vi "Flatten to CSV Record.vi"(0 "row of strings":string[](array[string]), 1 "protected symbol (,)":string=",", 2 "item separator (empty - use protected symbol)":string, 5 "error in (no error)":errorcluster) -> (3 "can be indented?":bool, 4 "CSV record":string, 6 "error out":errorcluster)   [LabVIEW 2013, in "infolib.lvlib"]
doc: "Convert 1D array of ANSI strings into a single CSV record (row or column).\n\nThe output CSV record string is formatted in accordance with RFC-4180 (see <b>http://tools.ietf.org/html/rfc4180<\\b>). \n\nAll cells containing double quotes (0x22), CR (0x0D) , LF (0x0A) or the delimiter character will be enclosed in double quotes. All double quote characters within a cell will be escaped using a second double quote character.\n\nRev. 0.0 2014-02-20 Ryan Porter\n- First Draft\n\nRev 0.1 2014-10-30 Ryan Porter\n- Convert all CRLF and CR within a cell to LF\n- Changed end of record to CRLF for compatibility with Excel CSV import/export\n\nRev 0.2 2017-01-03 modified for infolib\n\nRev 0.3 2017-01-20 can generate also column vector"
uses:
  infolib.lvlib
panel:
  # "Flatten to CSV Record.vi\n\nConvert 1D array of ANSI strings into a single CSV record (row). The output CSV record string is formatted in accordance with RFC-4180 (see http://tools.ietf.org/html/rfc4180). \n\nAll cells containing double quotes (0x22), CR (0x0D) , LF (0x0A) or the delimiter character will be enclosed in double quotes. All double quote characters within a cell will be escaped using a second double quote character. A CRLF is appended to the end of the record."
  # "License: BSD (2-Clause) - http://opensource.org/licenses/BSD-2-Clause \n\nCopyright (c) 2014, Ryan Porter\nAll rights reserved."
  # "Robust CSV v1.1.0\n\nCopyright © 2014, Ryan Porter\nAll rights reserved.\n\nAuthor:\t Ryan Porter\nLAVA Name: Porter\nContact Info:\tContact via PM on lavag.org\n\nLabVIEW Versions:\nLV 2013 (Windows)\nLV 2012 (Windows)\nLV 8.6 (Windows)\n\nDependencies:\nLAVA Palette\n\nDescription:\nThis package contains VIs for reading and writing to CSV files that follow the CSV format outlined in RFC-4180 (see http://tools.ietf.org/html/rfc4180). Using this package, you can properly import CSV files that were exported from spreadsheet programs such as Microsoft Excel, Open Office or LibreOffice Calc as well as export CSV files that will be compatible with any program capable of interpreting CSV files.\n \nThis implementation of the CSV format is capable of handling escaped fields such as those containing commas (or other field delimiters), multiple lines, and double quotes.\n\nInstallation and instructions:\nInstall VIP package using JKI VI Package Manager.\n\nExamples:\n\"<LabVIEW>\\examples\\LAVA\\Robust CSV\\Robust CSV Example Usage.vi\"\tDemonstrates usage of the Read CSV and Write CSV file.\n\nKnown Issues:\nnone\n\nAcknowledgements:\nPhillip Brooks: \"Parse CSV String.vi\" is a modified version of his \"CSV Data File Parser.vi\". His method of parsing the CSV string was much more efficient than my original implementation.\n\nVersion History:\nv1.0.0: Initial release of the code.\nv1.0.1: Modified \"Flatten to CSV Record.vi\" to play nice with Excel CSV import when multi-line cells are present.\nv1.1.0: Moved to LAVA palette & built to VI package file.\n\nLicense:\nDistributed under the BSD 2-Clause (http://opensource.org/licenses/BSD-2-Clause)\nSee link for a full description of the license.\n\nSupport:\nIf you have any problems with this code or want to suggest features go to lavag.org and Navigate to LAVA > Resources > Code Repository (Certified) and\nsearch for the \"Robust CSV\" support page. Or try this link: http://lavag.org/files/file/239-robust-csv/\n\nDistribution:\nThis code was downloaded from the LAVA Code Repository found at lavag.org"
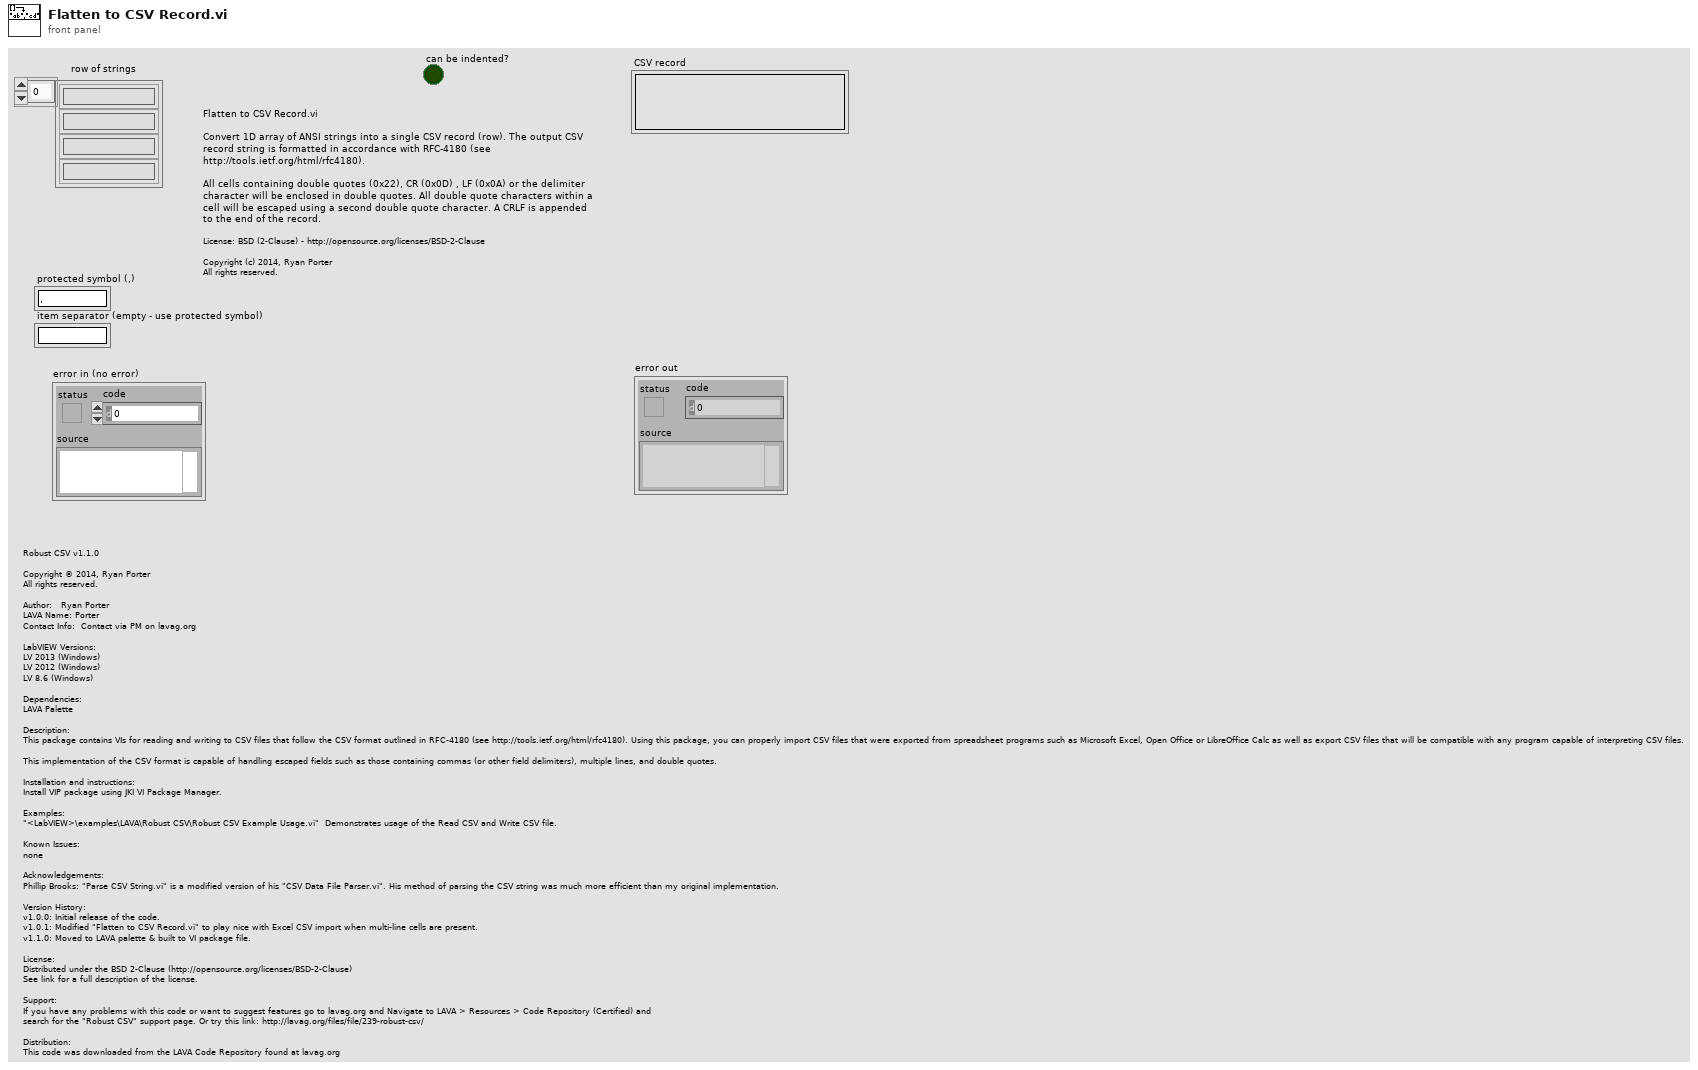
[diagram p1: front panel]
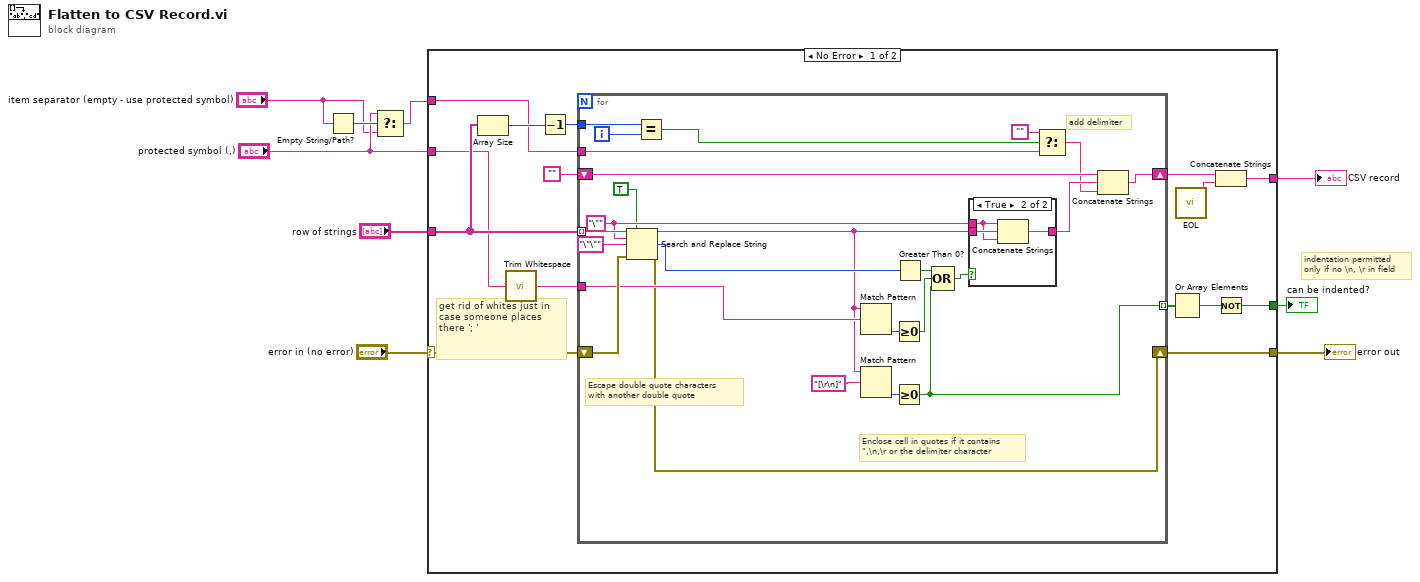
[diagram p0: block diagram]
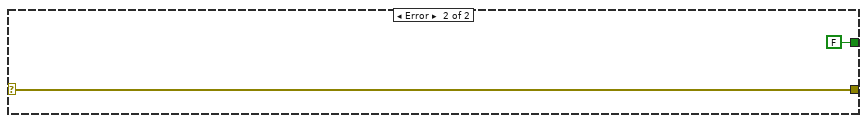
[diagram p3: hidden frame]
diagram:
  # "indentation permitted\nonly if no \\n, \\r in field"
  n1 = Empty String/Path?(string/path="item separator (empty - use protected symbol)") -> (empty?=w4:bool)
  n2 = Select(t="protected symbol (,)", s=w4, f="item separator (empty - use protected symbol)") -> (s? t:f=w1:string)
  n3 = case shown="No Error" "error in (no error)" {
    selector: "error in (no error)" -> [w18 w55]
    tunnel: "row of strings" -> [w22 _]
    tunnel: "protected symbol (,)" -> [w15 _]
    tunnel: [w19 _] -> w8
    tunnel: [w17 w55] -> w6
    tunnel: [w12 FALSE] -> w5
    tunnel: w1 -> [w10 _]
    frame No Error {
      # "get rid of whites just in case someone places there '; '"
      n4 = Array Size(array=w22) -> (size(s)=w21:i32)
      n5 = call <vilib>:"Trim Whitespace.vi"("string"=w15) -> ("trimmed string"=w11:string)  [unwired: 1 in]
      n6 = Decrement(x=w21) -> (x-1=w23:i32)
      n7 = for {
        tunnel: w22 -> [w49] mode=indexing
        shift-right: [w46] -> w20
        shift-left: "" -> [w45]
        tunnel: w10 -> [w40]
        tunnel: w23 -> [w37]
        shift-right: [w28] -> w17
        shift-left: w18 -> [w34]
        tunnel: [w25] -> w16 mode=indexing
        tunnel: w11 -> [w29]
        i -> [w42]
        w47 = "\"" ("search string")
        # "Escape double quote characters\nwith another double quote"
        # "Enclose cell in quotes if it contains\n\",\\n,\\r or the delimiter character"
        # "add delimiter"
        n8 = Search and Replace String(replace all?=TRUE ("replace all? (F)"), input string=w49, search string=w47, replace string="\"\"" ("replace string (\"\")"), error in=w34) -> (result string=w27:string, number of replacements=w36:i32, error out=w28:errorcluster)  [unwired: 4 out]
        n9 = Equal?(x=w37, y=w42) -> (x = y?=w41:bool)
        n10 = Match Pattern(string=w27, regular expression=w29) -> (offset past match=w43:i32)  [unwired: 4 out]
        n11 = Match Pattern(string=w27, regular expression="[\r\n]") -> (offset past match=w31:i32)  [unwired: 4 out]
        n12 = Greater Or Equal To 0?(x=w43) -> (x >= 0?=w26:bool)
        n13 = Greater Or Equal To 0?(x=w31) -> (x >= 0?=w25:bool)
        n14 = Greater Than 0?(x=w36) -> (x > 0?=w32:bool)
        n15 = Compound Arithmetic op=OR(w32, w26, w25) -> (w35:bool)
        n16 = case shown="True" w35 {
          tunnel: w27 -> [w50 w53]
          tunnel: w47 -> [_ w52]
          tunnel: [w50 w51] -> w44
          frame False {
          }
          frame True {
            n17 = Concatenate Strings(w52, w53, w52) -> (w51:string)
          }
        }
        n18 = Select(t="", s=w41, f=w40) -> (s? t:f=w38:string)
        n19 = Concatenate Strings(w45, w44, w38) -> (w46:string)
      }
      n20 = Or Array Elements(Boolean array=w16) -> (logical OR=w13:bool)
      n21 = call "EOL.vi"() -> ("eol"=w14:string)  [unwired: 11 in]
      n22 = Concatenate Strings(w20, w14) -> (w19:string)
      n23 = Not(x=w13) -> (.not. x?=w12:bool)
    }
    frame Error {
    }
  }
  "CSV record" <- w8
  "error out" <- w6
  "can be indented?" <- w5
